vi "SLSC CD Schema Path.vi"() -> (2 "SLSC CD Schema Path":string)   [LabVIEW 2017, in "VeriStand SLSC Scripting.lvlib"]
uses:
  VeriStand SLSC Scripting.lvlib
  NationalInstruments.VeriStand.SystemStorage
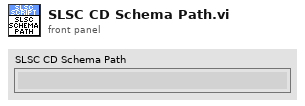
[diagram p1: front panel]
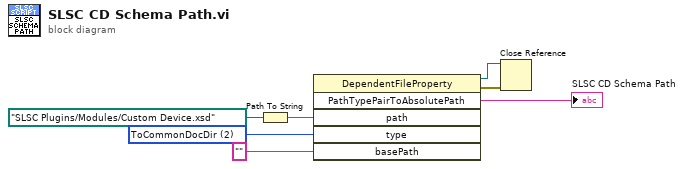
[diagram p0: block diagram]
diagram:
  w6 = 2 items=["Absolute", "Relative", "ToCommonDocDir", "ToApplicationDataDir"] ("type")
  n1 = Path To String(path=path "SLSC Plugins/Modules/Custom Device.xsd") -> (string=w3:string)
  n2 = invoke class="DependentFileProperty" method="PathTypePairToAbsolutePath"("path"=w3, "type"=w6, "basePath"="") -> (reference out=w1:refnum<k24>, error out=w2:errorcluster, "PathTypePairToAbsolutePath"=→"SLSC CD Schema Path":string)  [unwired: 3 in, 3 out]
  n3 = Close Reference(reference=w1, error in (no error)=w2) -> ()  [unwired: 1 out]
